vi "AnalyzeData.vi"(8 "error in (no error)":errorcluster, 11 "Queries":T1 {"Object Type" items=["File", "Channel Group", "Channel"]; "Operator" items=["=", "<>", ">", "<", ">=", "<=", "#"]}) -> (0 "error out":errorcluster, 3 "Refnum out":T4)   [LabVIEW 2014]
uses:
  <vilib>/DataFinder/NI_DataFinder Toolkit.lvlib
  <vilib>/DataFinder/Create Query (String).vi
  <vilib>/DataFinder/Create Query (Numeric).vi
  <vilib>/userdefined/DFQuery.ctl
  <vilib>/userdefined/NI_DataFinder Controls.lvlib
  <vilib>/DataFinder/DataTypes/comparison operator.ctl
  <vilib>/DataFinder/DataTypes/object type.ctl
  Controls/Query.ctl
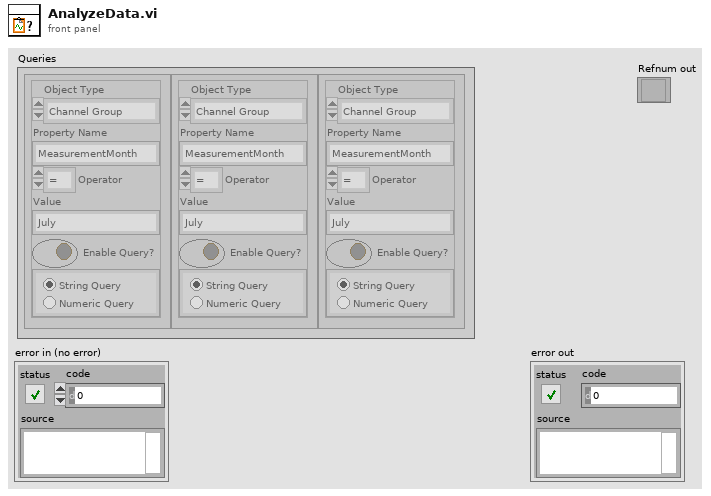
[diagram p1: front panel]
types:
  T1 = typedef "Query.ctl" = cluster{"Object Type":T2, "Property Name":string, "Operator":T3, "Value":string, "Enable Query?":bool, "Radio Buttons":enum32{"Radio Selection 1", "Radio Selection 2"}}[]
  T2 = typedef "NI_DataFinder Toolkit.lvlib/object type.ctl" = u16
  T3 = typedef "NI_DataFinder Toolkit.lvlib/comparison operator.ctl" = u16
  T4 = typedef "NI_DataFinder Controls.lvlib/DFQuery.ctl" = refnum<k20>
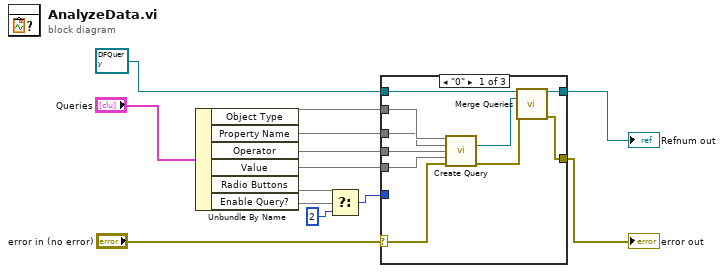
[diagram p0: block diagram]
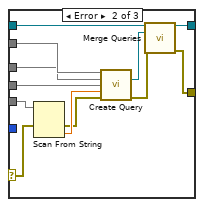
[diagram p2: hidden frame]
diagram:
  n1 = Unbundle By Name("Queries") -> ("Object Type"=w7, "Property Name"=w6, "Operator"=w5, "Value"=w8, "Radio Buttons"=w3, "Enable Query?"=w4)
  n2 = Select(t=w3, s=w4, f=2) -> (s? t:f=w1:i32)
  n3 = case shown="\"0\"" "error in (no error)" {
    selector: "error in (no error)" -> [w14 w25 w36]
    tunnel: w8 -> [w23 w27 _]
    tunnel: w7 -> [w22 w35 _]
    tunnel: w6 -> [w21 w34 _]
    tunnel: w5 -> [w20 w33 _]
    tunnel: T4 refnum ("query reference out") -> [w17 w30 w37]
    tunnel: [w16 w29 w37] -> w12
    tunnel: [w15 w28 w36] -> w11
    tunnel: w1 -> [_ _ _]
    frame No Error {
      n4 = call-poly <vilib>:"Create Query.vi"("object type"=w22, "property name"=w21, "comparison operator (=)"=w20, "value"=w23, "error in (no error)"=w14) -> ("query reference out"=w19:T4, "error out"=w18:errorcluster)  [unwired: 9 out]
      n5 = call <vilib>:"Merge Queries.vi"("query reference in 1"=w17, "query reference in 2"=w19, "error in (no error)"=w18) -> ("query reference out"=w16:T4, "error out"=w15:errorcluster)  [unwired: 2 in, 9 out]
    }
    frame Error {
      n6 = Scan From String(input string=w27, error in=w25) -> (error out=w24:errorcluster, output 1=w26:dbl)  [unwired: 3 in, 2 out]
      n7 = call-poly <vilib>:"Create Query.vi"("object type"=w35, "property name"=w34, "comparison operator (=)"=w33, "value"=w26, "error in (no error)"=w24) -> ("query reference out"=w32:T4, "error out"=w31:errorcluster)  [unwired: 9 out]
      n8 = call <vilib>:"Merge Queries.vi"("query reference in 1"=w30, "query reference in 2"=w32, "error in (no error)"=w31) -> ("query reference out"=w29:T4, "error out"=w28:errorcluster)  [unwired: 2 in, 9 out]
    }
    frame Error {
    }
  }
  "Refnum out" <- w12
  "error out" <- w11
